vi "Read Simple Sequencer Configuration.vi"(8 "error in (no error)":errorcluster, 11 "Simple Sequencer in":refnum<class "Simple Sequencer.lvclass">) -> (0 "error out":errorcluster, 2 "Configuration":T1, 3 "Simple Sequencer out":refnum<class "Simple Sequencer.lvclass">)   [LabVIEW 2018, in "Simple Sequencer.lvclass"]
uses:
  Simple Sequencer.lvclass
  C:/github/2018/LabActor/Template Module/Template Module.lvclass
  Simple Sequencer Configuration.ctl
  Template Module/Template Module.lvclass/Template Module.ctl
  Template Module/Read Configuration.vi
panel:
  # "Primary sequence"
  # "Secondary sequence"
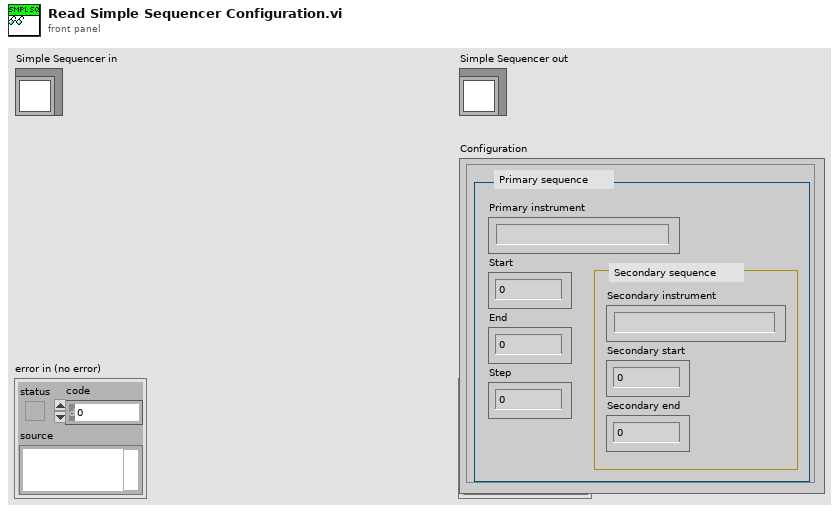
[diagram p1: front panel]
types:
  T1 = typedef "Simple Sequencer Configuration.ctl" = cluster{"Primary instrument":string, "Secondary instrument":string, "Start":dbl, "End":dbl, "Step":dbl, "Secondary start":dbl, "Secondary end":dbl}
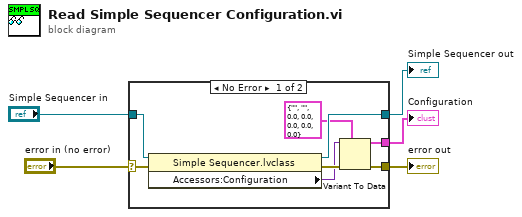
[diagram p0: block diagram]
diagram:
  n1 = case shown="No Error" "error in (no error)" {
    selector: "error in (no error)" -> [w13 w14]
    tunnel: [w9 w14] -> w4
    tunnel: [w10 w15] -> w2
    tunnel: "Simple Sequencer in" -> [w11 w15]
    tunnel: [w7 _] -> w1
    frame No Error {
      n2 = property class="Simple Sequencer.lvclass"(reference=w11, error in=w13) -> (reference out=w10:refnum<class "Simple Sequencer.lvclass">, error out=w12:errorcluster, "Accessors:Configuration"=w8:variant)
      n3 = Variant To Data(error in=w12, type=T1 {"Primary instrument"="", "Secondary instrument"="", "Start"=0.0, "End"=0.0, "Step"=0.0, "Secondary start"=0.0, "Secondary end"=0.0} ("Configuration"), Variant=w8) -> (data=w7:T1, error out=w9:errorcluster)
    }
    frame Error {
    }
  }
  "error out" <- w4
  "Simple Sequencer out" <- w2
  "Configuration" <- w1
